vi "BCU诊断标定.vi"(8 "CAN端口":u16(ring), 9 "设备索引号":u16(ring), 10 "CAN卡类型":u32(ring)=21, 11 "Myindex":dbl=1.0) -> (3 "成功":bool)   [LabVIEW 2013] (continued)
                tunnel: w6103 -> [w6106 w6114]
                frame #0 {
                  n4263 = dll-call lib="PTH1abs FBluewave New EnergySVN_WorkAutoTest_TestStandtrunkAutoTest_TestStandDriverZlgCanBHN01è¯»ååæ°data\nkerneldlls\nusbcan.dll" fn="VCI_ClearBuffer"("DeviceType"=w6108, "DeviceInd"=w6107, "CANInd"=w6106) -> (error out=w6109:errorcluster)  [unwired: 4 in, 4 out]
                  n4264 = call <vilib>:"Clear Errors.vi"("error in (no error)"=w6109) -> ()  [unwired: 6 in, 1 out]
                }
                frame #1 {
                  w6113 = u8 137 ("命令")
                  w6112 = u32 1 ("命令序号")
                  n4265 = local read "从板板号"() -> (w6110:u8)
                  n4266 = local write "命令"(w6113) -> ()
                  n4267 = call "多帧发送机制(EV05).vi"("can卡类型"=w6116, "设备索引号"=w6115, "CAN端口"=w6114, "命令"=w6113, "板号"=w6110, "命令序号"=w6112, "输入数据"=dbl[] [0.0]) -> ()  [unwired: 2 in, 11 out]
                  n4268 = local write "命令序号"(w6112) -> ()
                }
              }
            }
            frame #1 {
              n4269 = while {
                tunnel: [w6118] -> w6117
                i -> [w6123]
                stop <- w6120 stop-if-true
                n4270 = global read "EV05全局变量1.vi" "写入超时"() -> (w6118:bool)
                n4271 = Greater Or Equal?(x=w6123, y=25) -> (x >= y?=w6121:bool)
                n4272 = Or(x=w6118, y=w6121) -> (x .or. y?=w6120:bool)
                n4273 = Wait Until Next ms Multiple(millisecond multiple=u32 100 ("毫秒倍数")) -> ()  [unwired: 1 out]
              }
            }
            frame #2 {
              n4274 = case shown="假" w6124 {
                frame False {
                  n4275 = control-ref of="结果"() -> (w6126:refnum<vi>)
                  n4276 = Concatenate Strings("项目软件版本" ("字符串"), "     读取失败" ("字符串")) -> (w6129:string)
                  n4277 = Build Array(w6129) -> (w6128:string[])
                  n4278 = call "表格编辑(版本读取).vi"("新元素/子数组"=w6128, "活动单元格:单元格背景色"=u32 16740749, "MCListbox引用句柄"=w6126) -> ()  [unwired: 9 out]
                }
                frame True {
                }
              }
              n4279 = call <vilib>:"Unset Busy.vi"() -> ()  [unwired: 2 in, 10 out]
            }
          }
        }
        frame "读取故障状态" {
          n4280 = stacked-sequence {
            seq-local: [_ w6155 _] -> [_ _ w6162]
            frame #0 {
              n4281 = local read "设备索引号"() -> (w6132:u16)
              n4282 = local read "CAN卡类型"() -> (w6133:u32)
              n4283 = local read "CAN端口"() -> (w6131:u16)
              n4284 = stacked-sequence {
                tunnel: w6133 -> [w6136 w6145]
                tunnel: w6132 -> [w6135 w6144]
                tunnel: w6131 -> [w6134 w6143]
                frame #0 {
                  n4285 = dll-call lib="PTH1abs FBluewave New EnergySVN_WorkAutoTest_TestStandtrunkAutoTest_TestStandDriverZlgCanBHN01è¯»ååæ°data\nkerneldlls\nusbcan.dll" fn="VCI_ClearBuffer"("DeviceType"=w6136, "DeviceInd"=w6135, "CANInd"=w6134) -> (error out=w6137:errorcluster)  [unwired: 4 in, 4 out]
                  n4286 = call <vilib>:"Clear Errors.vi"("error in (no error)"=w6137) -> ()  [unwired: 6 in, 1 out]
                }
                frame #1 {
                  n4287 = local read "从板板号 2"() -> (w6138:u8)
                  n4288 = case shown="1..30" w6138 {
                    tunnel: [u8 133 ("命令") u8 4 ("命令")] -> w6142
                    frame 0, Default {
                    }
                    frame 1..30 {
                    }
                  }
                  n4289 = local read "状态选择"() -> (w6140:T18)
                  n4290 = local write "命令"(w6142) -> ()
                  n4291 = case shown="\"预充电故障,继电器驱动故障\"" w6140 {
                    tunnel: [1 2 3 4 5 6 7] -> w6139
                    frame "电压,内总电压,外总电压,温度,电流,绝缘,系统时钟,充电均衡,放电均衡", Default {
                    }
                    frame "CPU,CPU内部EE存储器,CPU内部FLASH,内部EE存储器,45db存储器" {
                    }
                    frame "CAN检测故障" {
                    }
                    frame "软件故障" {
                    }
                    frame "RS485,RS232检测故障" {
                    }
                    frame "DI,DO,AI,AO检测故障" {
                    }
                    frame "预充电故障,继电器驱动故障" {
                    }
                  }
                  n4292 = call "多帧发送机制(EV05).vi"("can卡类型"=w6145, "设备索引号"=w6144, "CAN端口"=w6143, "命令"=w6142, "板号"=w6138, "命令序号"=w6139, "输入数据"=dbl[] [0.0]) -> ()  [unwired: 2 in, 11 out]
                  n4293 = local write "命令序号"(w6139) -> ()
                }
              }
            }
            frame #1 {
              n4294 = while {
                tunnel: [w6156] -> w6155
                i -> [w6161]
                stop <- w6158 stop-if-true
                n4295 = global read "EV05全局变量1.vi" "写入超时"() -> (w6156:bool)
                n4296 = Greater Or Equal?(x=w6161, y=25) -> (x >= y?=w6159:bool)
                n4297 = Or(x=w6156, y=w6159) -> (x .or. y?=w6158:bool)
                n4298 = Wait Until Next ms Multiple(millisecond multiple=u32 100 ("毫秒倍数")) -> ()  [unwired: 1 out]
              }
            }
            frame #2 {
              n4299 = case shown="真" w6162 {
                frame False {
                  n4300 = Concatenate Strings("故障信息" ("字符串"), "     读取失败" ("字符串")) -> (w6164:string)
                  n4301 = One Button Dialog(message=w6164, button name ("OK")="确定" ("按钮名称（“确定”）")) -> ()  [unwired: 1 out]
                }
                frame True {
                  n4302 = One Button Dialog(message="故障信息读取完成" ("字符串"), button name ("OK")="确定" ("按钮名称（“确定”）")) -> ()  [unwired: 1 out]
                }
              }
              n4303 = call <vilib>:"Unset Busy.vi"() -> ()  [unwired: 2 in, 10 out]
            }
          }
        }
        frame "平台软件版本读取" {
          n4304 = stacked-sequence {
            seq-local: [_ w6184 _] -> [_ _ w6191]
            frame #0 {
              n4305 = local read "设备索引号"() -> (w6171:u16)
              n4306 = local read "CAN卡类型"() -> (w6172:u32)
              n4307 = local read "CAN端口"() -> (w6170:u16)
              n4308 = stacked-sequence {
                tunnel: w6172 -> [w6175 w6183]
                tunnel: w6171 -> [w6174 w6182]
                tunnel: w6170 -> [w6173 w6181]
                tunnel: u8 137 ("命令") -> [_ w6180]
                frame #0 {
                  n4309 = dll-call lib="PTH1abs FBluewave New EnergySVN_WorkAutoTest_TestStandtrunkAutoTest_TestStandDriverZlgCanBHN01è¯»ååæ°data\nkerneldlls\nusbcan.dll" fn="VCI_ClearBuffer"("DeviceType"=w6175, "DeviceInd"=w6174, "CANInd"=w6173) -> (error out=w6176:errorcluster)  [unwired: 4 in, 4 out]
                  n4310 = call <vilib>:"Clear Errors.vi"("error in (no error)"=w6176) -> ()  [unwired: 6 in, 1 out]
                }
                frame #1 {
                  w6179 = u32 2 ("命令序号")
                  n4311 = local read "从板板号"() -> (w6177:u8)
                  n4312 = local write "命令"(w6180) -> ()
                  n4313 = call "多帧发送机制(EV05).vi"("can卡类型"=w6183, "设备索引号"=w6182, "CAN端口"=w6181, "命令"=w6180, "板号"=w6177, "命令序号"=w6179, "输入数据"=dbl[] [0.0]) -> ()  [unwired: 2 in, 11 out]
                  n4314 = local write "命令序号"(w6179) -> ()
                }
              }
            }
            frame #1 {
              n4315 = while {
                tunnel: [w6185] -> w6184
                i -> [w6190]
                stop <- w6187 stop-if-true
                n4316 = global read "EV05全局变量1.vi" "写入超时"() -> (w6185:bool)
                n4317 = Greater Or Equal?(x=w6190, y=25) -> (x >= y?=w6188:bool)
                n4318 = Or(x=w6185, y=w6188) -> (x .or. y?=w6187:bool)
                n4319 = Wait Until Next ms Multiple(millisecond multiple=u32 100 ("毫秒倍数")) -> ()  [unwired: 1 out]
              }
            }
            frame #2 {
              n4320 = case shown="假" w6191 {
                frame False {
                  n4321 = control-ref of="结果"() -> (w6194:refnum<vi>)
                  n4322 = Concatenate Strings("平台软件版本" ("字符串"), "     读取失败" ("字符串")) -> (w6196:string)
                  n4323 = Build Array(w6196) -> (w6193:string[])
                  n4324 = call "表格编辑(版本读取).vi"("新元素/子数组"=w6193, "活动单元格:单元格背景色"=u32 16740749, "MCListbox引用句柄"=w6194) -> ()  [unwired: 9 out]
                }
                frame True {
                }
              }
              n4325 = call <vilib>:"Unset Busy.vi"() -> ()  [unwired: 2 in, 10 out]
            }
          }
        }
        frame "模块软件版本读取" {
          n4326 = local read "从板板号"() -> (w6198:u8)
          n4327 = local read "模块软件版本"() -> (w6199:T1)
          n4328 = case shown="\"全部读取\"" w6199 {
            selector: w6199 -> [w6200 w6244]
            tunnel: w6198 -> [_ w6243]
            frame "BCUMCAL", Default {
              n4329 = stacked-sequence {
                seq-local: [_ _ w6226 _] -> [_ _ _ w6233]
                tunnel: w6200 -> [_ w6206 _ w6234]
                frame #0 {
                  w6205 = FALSE ("写?")
                  n4330 = call <vilib>:"Set Busy.vi"("disable click? (T)"=FALSE) -> ()  [unwired: 3 in, 8 out]
                  n4331 = local write "写?"(w6205) -> ()
                  n4332 = global write "EV05全局变量1.vi" "流控帧 2"(TRUE ("流控帧 2")) -> ()
                  n4333 = global write "EV05全局变量1.vi" "写入超时"(w6205) -> ()
                  n4334 = local write "控制1"(TRUE ("控制1")) -> ()
                  n4335 = local write "消除"(TRUE ("消除")) -> ()
                }
                frame #1 {
                  n4336 = Quotient & Remainder(x=w6206, y=256) -> (x-y*floor(x/y)=w6207:i32, floor(x/y)=w6208:i32)
                  n4337 = Build Array(w6208, w6207, u8 0 ("板号")) -> (w6211:i32[])
                  n4338 = local read "设备索引号"() -> (w6213:u16)
                  n4339 = local read "CAN卡类型"() -> (w6214:u32)
                  n4340 = local read "CAN端口"() -> (w6212:u16)
                  n4341 = stacked-sequence {
                    tunnel: w6214 -> [w6217 w6225]
                    tunnel: w6213 -> [w6216 w6224]
                    tunnel: w6212 -> [w6215 w6223]
                    tunnel: w6211 -> [_ w6222]
                    frame #0 {
                      n4342 = dll-call lib="PTH1abs FBluewave New EnergySVN_WorkAutoTest_TestStandtrunkAutoTest_TestStandDriverZlgCanBHN01è¯»ååæ°data\nkerneldlls\nusbcan.dll" fn="VCI_ClearBuffer"("DeviceType"=w6217, "DeviceInd"=w6216, "CANInd"=w6215) -> (error out=w6218:errorcluster)  [unwired: 4 in, 4 out]
                      n4343 = call <vilib>:"Clear Errors.vi"("error in (no error)"=w6218) -> ()  [unwired: 6 in, 1 out]
                    }
                    frame #1 {
                      w6221 = u8 137 ("命令")
                      w6219 = u32 3 ("命令序号")
                      n4344 = local read "从板板号"() -> (w6220:u8)
                      n4345 = local write "命令"(w6221) -> ()
                      n4346 = call "多帧发送机制(EV05).vi"("can卡类型"=w6225, "设备索引号"=w6224, "CAN端口"=w6223, "命令"=w6221, "板号"=w6220, "命令序号"=w6219, "输入数据"=w6222) -> ()  [unwired: 2 in, 11 out]
                      n4347 = local write "命令序号"(w6219) -> ()
                    }
                  }
                }
                frame #2 {
                  n4348 = while {
                    tunnel: [w6227] -> w6226
                    i -> [w6232]
                    stop <- w6228 stop-if-true
                    n4349 = global read "EV05全局变量1.vi" "写入超时"() -> (w6227:bool)
                    n4350 = Greater Or Equal?(x=w6232, y=25) -> (x >= y?=w6229:bool)
                    n4351 = Or(x=w6227, y=w6229) -> (x .or. y?=w6228:bool)
                    n4352 = Wait Until Next ms Multiple(millisecond multiple=u32 100 ("毫秒倍数")) -> ()  [unwired: 1 out]
                  }
                }
                frame #3 {
                  n4353 = call <vilib>:"Unset Busy.vi"() -> ()  [unwired: 2 in, 10 out]
                  n4354 = case shown="假" w6233 {
                    tunnel: w6234 -> [w6236 _]
                    frame False {
                      n4355 = Number To Decimal String(number=w6236) -> (decimal integer string=w6237:string)  [unwired: 1 out]
                      n4356 = control-ref of="结果"() -> (w6238:refnum<vi>)
                      n4357 = Concatenate Strings("模块" ("字符串"), w6237, "     读取失败" ("字符串")) -> (w6241:string)
                      n4358 = Build Array(w6241) -> (w6240:string[])
                      n4359 = call "表格编辑(版本读取).vi"("新元素/子数组"=w6240, "活动单元格:单元格背景色"=u32 16740749, "MCListbox引用句柄"=w6238) -> ()  [unwired: 9 out]
                    }
                    frame True {
                    }
                  }
                }
              }
            }
            frame "全部读取" {
              n4360 = stacked-sequence {
                seq-local: [w6245 _] -> [_ w6283]
                tunnel: w6244 -> [_ w6285]
                tunnel: w6243 -> [w6246 w6284]
                frame #0 {
                  n4361 = stacked-sequence {
                    tunnel: w6246 -> [_ w6255 _]
                    tunnel: [_ _ w6275] -> w6245
                    frame #0 {
                      w6251 = FALSE ("写?")
                      n4362 = control-ref of="模块软件版本 2"() -> (w6249:refnum<vi>)
                      n4363 = call <vilib>:"Set Busy.vi"("disable click? (T)"=FALSE) -> ()  [unwired: 3 in, 8 out]
                      n4364 = local write "写?"(w6251) -> ()
                      n4365 = property class="MCListbox (严格)"(reference=w6249, "ItemNames"=string[][] []) -> ()  [unwired: 1 in, 2 out]
                      n4366 = global write "EV05全局变量1.vi" "写入超时"(w6251) -> ()
                      n4367 = local write "消除"(TRUE ("消除")) -> ()
                      n4368 = local write "控制1"(TRUE ("控制1")) -> ()
                      n4369 = global write "EV05全局变量1.vi" "流控帧 2"(TRUE ("流控帧 2")) -> ()
                      n4370 = local write "MODEL号"(u8[] [] ("MODEL号")) -> ()
                    }
                    frame #1 {
                      n4371 = local read "设备索引号"() -> (w6257:u16)
                      n4372 = local read "CAN卡类型"() -> (w6258:u32)
                      n4373 = local read "CAN端口"() -> (w6256:u16)
                      n4374 = stacked-sequence {
                        tunnel: w6258 -> [w6261 w6274]
                        tunnel: w6257 -> [w6260 w6273]
                        tunnel: w6256 -> [w6259 w6272]
                        tunnel: w6255 -> [_ w6264]
                        frame #0 {
                          n4375 = dll-call lib="PTH1abs FBluewave New EnergySVN_WorkAutoTest_TestStandtrunkAutoTest_TestStandDriverZlgCanBHN01è¯»ååæ°data\nkerneldlls\nusbcan.dll" fn="VCI_ClearBuffer"("DeviceType"=w6261, "DeviceInd"=w6260, "CANInd"=w6259) -> (error out=w6262:errorcluster)  [unwired: 4 in, 4 out]
                          n4376 = call <vilib>:"Clear Errors.vi"("error in (no error)"=w6262) -> ()  [unwired: 6 in, 1 out]
                        }
                        frame #1 {
                          w6270 = u8 137 ("命令")
                          w6268 = u32 3 ("命令序号")
                          n4377 = Quotient & Remainder(x=u8 0 ("板号"), y=256) -> (x-y*floor(x/y)=w6265:i32, floor(x/y)=w6266:i32)
                          n4378 = local write "命令"(w6270) -> ()
                          n4379 = Build Array(w6266, w6265, u8 0 ("板号")) -> (w6271:i32[])
                          n4380 = call "多帧发送机制(EV05).vi"("can卡类型"=w6274, "设备索引号"=w6273, "CAN端口"=w6272, "命令"=w6270, "板号"=w6264, "命令序号"=w6268, "输入数据"=w6271) -> ()  [unwired: 2 in, 11 out]
                          n4381 = local write "命令序号"(w6268) -> ()
                        }
                      }
                    }
                    frame #2 {
                      n4382 = while {
                        tunnel: [w6277] -> w6275
                        i -> [w6281]
                        stop <- w6278 stop-if-true
                        n4383 = local read "强制停止版本读取"() -> (w6276:bool)
                        n4384 = global read "EV05全局变量1.vi" "写入超时"() -> (w6277:bool)
                        n4385 = Greater Or Equal?(x=w6281, y=35) -> (x >= y?=w6279:bool)
                        n4386 = Compound Arithmetic op=OR(w6276, w6277, w6279) -> (w6278:bool)
                        n4387 = Wait Until Next ms Multiple(millisecond multiple=u32 100 ("毫秒倍数")) -> ()  [unwired: 1 out]
                      }
                    }
                  }
                }
                frame #1 {
                  n4388 = case shown="真" w6283 {
                    tunnel: w6285 -> [_ w6295]
                    tunnel: w6284 -> [_ w6294]
                    frame False {
                      n4389 = control-ref of="结果"() -> (w6287:refnum<vi>)
                      n4390 = Concatenate Strings("模块编号" ("字符串"), "读取失败" ("字符串")) -> (w6290:string)
                      n4391 = Build Array(w6290) -> (w6289:string[])
                      n4392 = call "表格编辑(版本读取).vi"("新元素/子数组"=w6289, "活动单元格:单元格背景色"=u32 16740749, "MCListbox引用句柄"=w6287) -> ()  [unwired: 9 out]
                      n4393 = call <vilib>:"Unset Busy.vi"() -> ()  [unwired: 11 in, 1 out]
                    }
                    frame True {
                      n4394 = local read "MODEL号"() -> (w6293:u8[])
                      n4395 = Array Size(array=w6293) -> (size(s)=w6292:i32)
                      n4396 = for {
                        tunnel: w6295 -> [_]
                        tunnel: w6294 -> [w6298]
                        tunnel: w6293 -> [w6297] mode=indexing
                        tunnel: w6292 -> [w6296]
                        i -> [w6300]
                        n4397 = Increment(x=w6300) -> (x+1=w6299:i32)
                        n4398 = stacked-sequence {
                          seq-local: [_ _ _ w6327 _ _] -> [_ _ _ _ w6336 _]
                          seq-local: [_ w6306 _ _ _ _] -> [_ _ _ _ w6335 _]
                          tunnel: w6299 -> [_ _ _ _ _ w6347]
                          tunnel: w6297 -> [_ w6306 _ _ _ _]
                          tunnel: w6298 -> [_ w6307 _ _ _ _]
                          tunnel: w6296 -> [_ _ _ _ _ w6345]
                          frame #0 {
                            w6302 = FALSE ("写?")
                            n4399 = call <vilib>:"Set Busy.vi"("disable click? (T)"=FALSE) -> ()  [unwired: 3 in, 8 out]
                            n4400 = local write "写?"(w6302) -> ()
                            n4401 = global write "EV05全局变量1.vi" "写入超时"(w6302) -> ()
                            n4402 = global write "EV05全局变量1.vi" "流控帧 2"(TRUE ("流控帧 2")) -> ()
                            n4403 = local write "控制1"(TRUE ("控制1")) -> ()
                            n4404 = local write "消除"(TRUE ("消除")) -> ()
                          }
                          frame #1 {
                            n4405 = local read "设备索引号"() -> (w6309:u16)
                            n4406 = local read "CAN卡类型"() -> (w6310:u32)
                            n4407 = local read "CAN端口"() -> (w6308:u16)
                            n4408 = stacked-sequence {
                              tunnel: w6310 -> [w6313 w6326]
                              tunnel: w6309 -> [w6312 w6325]
                              tunnel: w6308 -> [w6311 w6324]
                              tunnel: w6307 -> [_ w6316]
                              tunnel: w6306 -> [_ w6315]
                              frame #0 {
                                n4409 = dll-call lib="PTH1abs FBluewave New EnergySVN_WorkAutoTest_TestStandtrunkAutoTest_TestStandDriverZlgCanBHN01è¯»ååæ°data\nkerneldlls\nusbcan.dll" fn="VCI_ClearBuffer"("DeviceType"=w6313, "DeviceInd"=w6312, "CANInd"=w6311) -> (error out=w6314:errorcluster)  [unwired: 4 in, 4 out]
                                n4410 = call <vilib>:"Clear Errors.vi"("error in (no error)"=w6314) -> ()  [unwired: 6 in, 1 out]
                              }
                              frame #1 {
                                w6322 = u8 137 ("命令")
                                w6320 = u32 3 ("命令序号")
                                n4411 = Quotient & Remainder(x=w6315, y=256) -> (x-y*floor(x/y)=w6317:i32, floor(x/y)=w6318:i32)
                                n4412 = local write "命令"(w6322) -> ()
                                n4413 = Build Array(w6318, w6317, u8 0 ("板号")) -> (w6323:i32[])
                                n4414 = call "多帧发送机制(EV05).vi"("can卡类型"=w6326, "设备索引号"=w6325, "CAN端口"=w6324, "命令"=w6322, "板号"=w6316, "命令序号"=w6320, "输入数据"=w6323) -> ()  [unwired: 2 in, 11 out]
                                n4415 = local write "命令序号"(w6320) -> ()
                              }
                            }
                          }
                          frame #2 {
                          }
                          frame #3 {
                            n4416 = while {
                              tunnel: [w6329] -> w6327
                              i -> [w6333]
                              stop <- w6330 stop-if-true
                              n4417 = local read "强制停止版本读取"() -> (w6328:bool)
                              n4418 = global read "EV05全局变量1.vi" "写入超时"() -> (w6329:bool)
                              n4419 = Greater Or Equal?(x=w6333, y=25) -> (x >= y?=w6331:bool)
                              n4420 = Compound Arithmetic op=OR(w6328, w6329, w6331) -> (w6330:bool)
                              n4421 = Wait Until Next ms Multiple(millisecond multiple=u32 100 ("毫秒倍数")) -> ()  [unwired: 1 out]
                            }
                          }
                          frame #4 {
                            n4422 = call <vilib>:"Unset Busy.vi"() -> ()  [unwired: 11 in, 1 out]
                            n4423 = case shown="假" w6336 {
                              tunnel: w6335 -> [w6338 _]
                              frame False {
                                n4424 = control-ref of="结果"() -> (w6340:refnum<vi>)
                                n4425 = Number To Decimal String(number=w6338) -> (decimal integer string=w6339:string)  [unwired: 1 out]
                                n4426 = Concatenate Strings("模块" ("字符串"), w6339, "     读取失败" ("字符串")) -> (w6343:string)
                                n4427 = Build Array(w6343) -> (w6342:string[])
                                n4428 = call "表格编辑(版本读取).vi"("新元素/子数组"=w6342, "活动单元格:单元格背景色"=u32 16740749, "MCListbox引用句柄"=w6340) -> ()  [unwired: 9 out]
                              }
                              frame True {
                              }
                            }
                          }
                          frame #5 {
                            n4429 = Equal?(x=w6345, y=w6347) -> (x = y?=w6346:bool)
                            n4430 = case shown="真" w6346 {
                              frame False {
                              }
                              frame True {
                                n4431 = control-ref of="模块软件版本 2"() -> (w6358:refnum<vi>)
                                n4432 = local read "模块版本名称"() -> (w6357:string[][])
                                n4433 = local read "模块版本值"() -> (w6353:string[][])
                                n4434 = control-ref of="结果"() -> (w6365:refnum<vi>)
                                n4435 = property class="MCListbox (严格)"(reference=w6358) -> ("ItemNames"=w6361:string[][])  [unwired: 1 in, 2 out]
                                n4436 = local read "从板板号"() -> (w6348:u8)
                                n4437 = Concatenate Strings("模块版本读取完成" ("字符串")) -> (w6368:string)
                                n4438 = Build Array(w6368) -> (w6367:string[])
                                n4439 = call "表格编辑(版本读取).vi"("新元素/子数组"=w6367, "活动单元格:单元格背景色"=u32 21937, "MCListbox引用句柄"=w6365) -> ()  [unwired: 9 out]
                                n4440 = Transpose 2D Array(2D array=w6361) -> (transposed array=w6362:string[][])
                                n4441 = local write "强制停止版本读取"(FALSE ("强制停止 2")) -> ()
                                n4442 = local read "模块个数"() -> (w6351:u8[])
                                n4443 = Index Array(array=w6362, index (row) #1=0 ("索引 (行)"), index (row) #2=1 ("索引 (行)")) -> (element #1=w6352:string[], element #2=w6354:string[])  [unwired: 2 in]
                                n4444 = Replace Array Subset(array=w6357, new element=w6352, index (row)=w6348) -> (w6356:string[][])  [unwired: 1 in]
                                n4445 = Replace Array Subset(array=w6353, new element=w6354, index (row)=w6348) -> (w6355:string[][])  [unwired: 1 in]
                                n4446 = local write "模块版本名称"(w6356) -> ()
                                n4447 = local write "模块版本值"(w6355) -> ()
                                n4448 = Array Size(array=w6352) -> (size(s)=w6349:i32)
                                n4449 = Replace Array Subset(array=w6351, new element=w6349, index=w6348) -> (w6350:u8[])
                                n4450 = local write "模块个数"(w6350) -> ()
                              }
                            }
                          }
                        }
                      }
                    }
                  }
                }
              }
            }
          }
        }
        frame "硬件版本读取" {
          n4451 = stacked-sequence {
            seq-local: [_ _ w6376 _] -> [_ _ _ w6383]
            frame #0 {
              w6372 = u8 137 ("命令")
              w6371 = u32 4 ("命令序号")
              n4452 = local read "设备索引号"() -> (w6374:u16)
              n4453 = local read "CAN卡类型"() -> (w6375:u32)
              n4454 = local read "CAN端口"() -> (w6373:u16)
              n4455 = local read "从板板号"() -> (w6369:u8)
              n4456 = local write "命令"(w6372) -> ()
              n4457 = call "多帧发送机制(EV05).vi"("can卡类型"=w6375, "设备索引号"=w6374, "CAN端口"=w6373, "命令"=w6372, "板号"=w6369, "命令序号"=w6371, "输入数据"=dbl[] [0.0]) -> ()  [unwired: 2 in, 11 out]
              n4458 = local write "命令序号"(w6371) -> ()
            }
            frame #1 {
            }
            frame #2 {
              n4459 = while {
                tunnel: [w6377] -> w6376
                i -> [w6382]
                stop <- w6378 stop-if-true
                n4460 = global read "EV05全局变量1.vi" "写入超时"() -> (w6377:bool)
                n4461 = Greater Or Equal?(x=w6382, y=25) -> (x >= y?=w6379:bool)
                n4462 = Or(x=w6377, y=w6379) -> (x .or. y?=w6378:bool)
                n4463 = Wait Until Next ms Multiple(millisecond multiple=u32 100 ("毫秒倍数")) -> ()  [unwired: 1 out]
              }
            }
            frame #3 {
              n4464 = case shown="假" w6383 {
                frame False {
                  n4465 = control-ref of="结果"() -> (w6385:refnum<vi>)
                  n4466 = Concatenate Strings("硬件版本" ("字符串"), "     读取失败" ("字符串")) -> (w6388:string)
                  n4467 = Build Array(w6388) -> (w6387:string[])
                  n4468 = call "表格编辑(版本读取).vi"("新元素/子数组"=w6387, "活动单元格:单元格背景色"=u32 16740749, "MCListbox引用句柄"=w6385) -> ()  [unwired: 9 out]
                }
                frame True {
                }
              }
              n4469 = call <vilib>:"Unset Busy.vi"() -> ()  [unwired: 2 in, 10 out]
            }
          }
        }
        frame "写配置文件" {
          n4470 = disable-structure shown="启用" {
            frame Enabled {
              n4471 = local read "主从选择"() -> (w6396:enum32{"主板", "从板"})
              n4472 = case shown="\"从板\"" w6396 {
                tunnel: [w6415 w6606] -> w6399
                tunnel: ["M0" w6612] -> w6397
                frame "主板", Default {
                  n4473 = stacked-sequence {
                    seq-local: [w6429 _ _ _ _ _ _] -> [_ w6458 _ _ _ _ _]
                    seq-local: [string[] ["电池额定容量", "电池实际容量", "SOC", "SOH", "车牌号", "配置文件版本", "产品编号", "系统时钟"] _ _ _ _ _ _] -> [_ w6453 _ _ _ _ _]
                    seq-local: [_ _ _ _ string[] ["风机开启温度", "风机关闭温度", "加热开启温度", "加热关闭温度", "风机开启温差", "风机关闭温差", "加热关闭温差"] _ _] -> [_ _ _ _ _ w6558 _]
                    seq-local: [_ _ _ _ w6539 _ _] -> [_ _ _ _ _ w6556 _]
                    tunnel: [w6430 _ _ _ _ _ _] -> w6417
                    tunnel: [_ w6460 _ _ _ _ _] -> w6414
                    tunnel: [_ _ w6484 _ _ _ _] -> w6413
                    tunnel: [_ _ _ w6511 _ _ _] -> w6412
                    tunnel: [_ _ _ _ _ w6559 _] -> w6411
                    tunnel: [_ _ _ _ _ _ w6576] -> w6410
                    frame #0 {
                      w6421 = string[] ["", "", "", "", "", "", "", "", "", "", "  "]
                      n4474 = control-ref of="项目信息"() -> (w6449:refnum<vi>)
                      n4475 = property class="Tbl (严格)"(reference=w6449) -> ("Value"=w6425:string[][])  [unwired: 1 in, 2 out]
                      n4476 = control-ref of="项目信息2"() -> (w6443:refnum<vi>)
                      n4477 = Index Array(array=w6425, index (col)=0 ("禁用的索引 (列)")) -> (element=w6426:string[])  [unwired: 1 in]
                      n4478 = property class="Clust (严格)"(reference=w6443) -> ("Value"=w6442:T9)  [unwired: 1 in, 2 out]
                      n4479 = Index Array(array=w6425, index (col)=1 ("禁用的索引 (列)")) -> (element=w6424:string[])  [unwired: 1 in]
                      n4480 = local read "从板个数"() -> (w6448:dbl)
                      n4481 = Number To Decimal String(number=w6448) -> (decimal integer string=w6447:string)  [unwired: 1 out]
                      n4482 = Insert Into Array(array=w6426, new element=w6421) -> (w6423:string[])  [unwired: 1 in]
                      n4483 = Insert Into Array(array=w6424, new element=w6421) -> (w6422:string[])  [unwired: 1 in]
                      n4484 = Unbundle(w6442) -> ("电池额定容量(A)"=w6441:dbl, "电池实际容量(A)"=w6440:dbl, "车架(牌)号"=w6438:string, "配置文件版本"=w6437:string, "SOH(%)"=w6432:dbl, "SOC(%)"=w6431:dbl, "产品编号"=w6436:string, "系统时钟"=w6435:string)  [unwired: 1 out]
                      n4485 = Build Array("从板个数" ("元素"), w6447) -> (w6444:string[])
                      n4486 = Build Array(w6423, w6422) -> (w6419:string[][])
                      n4487 = Transpose 2D Array(2D array=w6419) -> (transposed array=w6418:string[][])
                      n4488 = Build Array(w6441, w6440, w6431, w6432) -> (w6439:dbl[])
                      n4489 = Build Array(w6438, w6437, w6436, w6435) -> (w6433:string[])
                      n4490 = for {
                        tunnel: w6439 -> [w6451] mode=indexing
                        tunnel: [w6450] -> w6434 mode=indexing
                        n4491 = Format Into String(format string="%#f" ("格式字符串"), w6451) -> (resulting string=w6450:string)  [unwired: 2 in, 1 out]
                      }
                      n4492 = Insert Into Array(array=w6418, index (row)=0 ("索引 (行)"), new element=w6444) -> (w6430:string[][])  [unwired: 1 in]
                      n4493 = Insert Into Array(array=w6434, new element=w6433) -> (w6429:string[])  [unwired: 1 in]
                    }
                    frame #1 {
                      n4494 = control-ref of="一级故障"() -> (w6480:refnum<vi>)
                      n4495 = property class="Clust (严格)"(reference=w6480) -> ("Value"=w6479:T10)  [unwired: 1 in, 2 out]
                      n4496 = Unbundle(w6479) -> ("总电压过高"=w6478:dbl, "整组电压不均衡"=w6473:dbl, "SOC过高"=w6466:dbl, "单体电压过高"=w6469:dbl, "总电压过低"=w6477:dbl, "温度过高"=w6476:dbl, "温度过低"=w6475:dbl, "单组电压不均衡"=w6474:dbl, "整组温度不均衡"=w6471:dbl, "单组温度不均衡"=w6472:dbl, "单体电压过低"=w6470:dbl, "充电电流过高"=w6468:dbl, "放电电流过高"=w6467:dbl, "SOC过低"=w6465:dbl, "内阻过大"=w6464:dbl, "极柱温度过高"=w6463:dbl, "SOH过低"=w6462:dbl)
                      n4497 = Build Array(w6478, w6477, w6476, w6475, w6474, w6473, w6472, w6471, w6469, w6470, w6468, w6467, w6466, w6465, w6464, w6463, w6462) -> (w6461:dbl[])
                      n4498 = for {
                        tunnel: w6461 -> [w6482] mode=indexing
                        tunnel: [w6481] -> w6457 mode=indexing
                        n4499 = Format Into String(format string="%#f" ("格式字符串"), w6482) -> (resulting string=w6481:string)  [unwired: 2 in, 1 out]
                      }
                      n4500 = Insert Into Array(array=w6458, new element=w6457) -> (w6456:string[])  [unwired: 1 in]
                      n4501 = Insert Into Array(array=w6453, new element=string[] ["总电压过高一级", "总电压过低一级", "温度过高一级", "温度过低一级", "单组电压不均衡一级", "整组电压不均衡一级", "单组温度不均衡一级", "整组温度不均衡一级", "单体电压过高一级", "单体电压过低一级", "充电电流过高一级", "放电电流过高一级", "SOC过高一级", "SOC过低一级", "内阻过大一级", "极柱温度过高一级", "SOH过低一级"]) -> (w6455:string[])  [unwired: 1 in]
                      n4502 = Build Array(w6455, w6456) -> (w6454:string[][])
                      n4503 = Transpose 2D Array(2D array=w6454) -> (transposed array=w6460:string[][])
                    }
                    frame #2 {
                      n4504 = control-ref of="一级故障 2"() -> (w6485:refnum<vi>)
                      n4505 = property class="Clust (严格)"(reference=w6485) -> ("Value"=w6507:T10)  [unwired: 1 in, 2 out]
                      n4506 = Unbundle(w6507) -> ("总电压过高"=w6506:dbl, "整组电压不均衡"=w6501:dbl, "SOC过高"=w6494:dbl, "单体电压过高"=w6497:dbl, "总电压过低"=w6505:dbl, "温度过高"=w6504:dbl, "温度过低"=w6503:dbl, "单组电压不均衡"=w6502:dbl, "整组温度不均衡"=w6499:dbl, "单组温度不均衡"=w6500:dbl, "单体电压过低"=w6498:dbl, "充电电流过高"=w6496:dbl, "放电电流过高"=w6495:dbl, "SOC过低"=w6493:dbl, "内阻过大"=w6492:dbl, "极柱温度过高"=w6491:dbl, "SOH过低"=w6490:dbl)
                      n4507 = Build Array(w6506, w6505, w6504, w6503, w6502, w6501, w6500, w6499, w6497, w6498, w6496, w6495, w6494, w6493, w6492, w6491, w6490) -> (w6489:dbl[])
                      n4508 = for {
                        tunnel: w6489 -> [w6509] mode=indexing
                        tunnel: [w6508] -> w6488 mode=indexing
                        n4509 = Format Into String(format string="%#f" ("格式字符串"), w6509) -> (resulting string=w6508:string)  [unwired: 2 in, 1 out]
                      }
                      n4510 = Build Array(string[] ["总电压过高二级", "总电压过低二级", "温度过高二级", "温度过低二级", "单组电压不均衡二级", "整组电压不均衡二级", "单组温度不均衡二级", "整组温度不均衡二级", "单体电压过高二级", "单体电压过低二级", "充电电流过高二级", "放电电流过高二级", "SOC过高二级", "SOC过低二级", "内阻过大二级", "极柱温度过高二级", "SOH过低二级"], w6488) -> (w6486:string[][])
                      n4511 = Transpose 2D Array(2D array=w6486) -> (transposed array=w6484:string[][])
                    }
                    frame #3 {
                      n4512 = control-ref of="一级故障 3"() -> (w6512:refnum<vi>)
                      n4513 = property class="Clust (严格)"(reference=w6512) -> ("Value"=w6534:T10)  [unwired: 1 in, 2 out]
                      n4514 = Unbundle(w6534) -> ("总电压过高"=w6533:dbl, "整组电压不均衡"=w6528:dbl, "SOC过高"=w6521:dbl, "单体电压过高"=w6524:dbl, "总电压过低"=w6532:dbl, "温度过高"=w6531:dbl, "温度过低"=w6530:dbl, "单组电压不均衡"=w6529:dbl, "整组温度不均衡"=w6526:dbl, "单组温度不均衡"=w6527:dbl, "单体电压过低"=w6525:dbl, "充电电流过高"=w6523:dbl, "放电电流过高"=w6522:dbl, "SOC过低"=w6520:dbl, "内阻过大"=w6519:dbl, "极柱温度过高"=w6518:dbl, "SOH过低"=w6517:dbl)
                      n4515 = Build Array(w6533, w6532, w6531, w6530, w6529, w6528, w6527, w6526, w6524, w6525, w6523, w6522, w6521, w6520, w6519, w6518, w6517) -> (w6516:dbl[])
                      n4516 = for {
                        tunnel: w6516 -> [w6536] mode=indexing
                        tunnel: [w6535] -> w6515 mode=indexing
                        n4517 = Format Into String(format string="%#f" ("格式字符串"), w6536) -> (resulting string=w6535:string)  [unwired: 2 in, 1 out]
                      }
                      n4518 = Build Array(string[] ["总电压过高三级", "总电压过低三级", "温度过高三级", "温度过低三级", "单组电压不均衡三级", "整组电压不均衡三级", "单组温度不均衡三级", "整组温度不均衡三级", "单体电压过高三级", "单体电压过低三级", "充电电流过高三级", "放电电流过高三级", "SOC过高三级", "SOC过低三级", "内阻过大三级", "极柱温度过高三级", "SOH过低三级"], w6515) -> (w6513:string[][])
                      n4519 = Transpose 2D Array(2D array=w6513) -> (transposed array=w6511:string[][])
                    }
                    frame #4 {
                      n4520 = control-ref of="加热控制参数"() -> (w6549:refnum<vi>)
                      n4521 = property class="Clust (严格)"(reference=w6549) -> ("Value"=w6548:T11)  [unwired: 1 in, 2 out]
                      n4522 = Unbundle(w6548) -> ("风机开启温度"=w6547:dbl, "风机关闭温度"=w6546:dbl, "加热开启温度"=w6545:dbl, "加热关闭温度"=w6544:dbl, "风机开启温差"=w6543:dbl, "风机关闭温差"=w6542:dbl, "加热关闭温差"=w6538:dbl)
                      n4523 = Build Array(w6547, w6546, w6545, w6544, w6543, w6542, w6538) -> (w6541:dbl[])
                      n4524 = for {
                        tunnel: w6541 -> [w6551] mode=indexing
                        tunnel: [w6550] -> w6539 mode=indexing
                        n4525 = Format Into String(format string="%#f" ("格式字符串"), w6551) -> (resulting string=w6550:string)  [unwired: 2 in, 1 out]
                      }
                    }
                    frame #5 {
                      n4526 = control-ref of="充电控制参数"() -> (w6569:refnum<vi>)
                      n4527 = property class="Clust (严格)"(reference=w6569) -> ("Value"=w6571:T12)  [unwired: 1 in, 2 out]
                      n4528 = Unbundle(w6571) -> ("最大允许单体电压"=w6568:dbl, "最大允许总电压"=w6567:dbl, "最小允许单体电压"=w6566:dbl, "最大允许充电电流"=w6565:dbl, "最小允许充电电流"=w6564:dbl, "最大允许充电温度"=w6563:dbl, "最小允许充电温度"=w6562:dbl, "电流步长"=w6561:dbl)
                      n4529 = Build Array(w6568, w6567, w6566, w6565, w6564, w6563, w6562, w6561) -> (w6570:dbl[])
                      n4530 = for {
                        tunnel: w6570 -> [w6573] mode=indexing
                        tunnel: [w6572] -> w6555 mode=indexing
                        n4531 = Format Into String(format string="%#f" ("格式字符串"), w6573) -> (resulting string=w6572:string)  [unwired: 2 in, 1 out]
                      }
                      n4532 = Insert Into Array(array=w6556, new element=w6555) -> (w6554:string[])  [unwired: 1 in]
                      n4533 = Insert Into Array(array=w6558, new element=string[] ["最大允许单体电压", "最大允许总电压", "最小允许单体电压", "最大允许充电电流", "最小允许充电电流", "最大允许充电温度", "最小允许充电温度", "电流步长"]) -> (w6553:string[])  [unwired: 1 in]
                      n4534 = Build Array(w6553, w6554) -> (w6560:string[][])
                      n4535 = Transpose 2D Array(2D array=w6560) -> (transposed array=w6559:string[][])
                    }
                    frame #6 {
                      n4536 = control-ref of="电池信息"() -> (w6597:refnum<vi>)
                      n4537 = property class="Clust (严格)"(reference=w6597) -> ("Value"=w6600:T13)  [unwired: 1 in, 2 out]
                      n4538 = Unbundle(w6600) -> ("电池串联"=w6596:dbl, "电池并联"=w6595:dbl, "累计放电总安时"=w6593:dbl, "电池包额定容量"=w6592:dbl, "电池包额定能量(kWh)"=w6591:dbl, "电池包额定总电压"=w6590:dbl, "累计充电总安时"=w6594:dbl, "电池充满次数"=w6589:dbl, "电池放空次数"=w6588:dbl, "电池充电次数"=w6587:dbl, "电池生产日期"=w6585:string, "电池厂家"=w6584:string, "电池类型"=w6583:string, "电池包组号"=w6582:string, "电池包产权标识"=w6581:string, "电池应用车型"=w6580:string, "实际容量"=w6575:dbl)
                      n4539 = Build Array(w6585, w6584, w6583, w6582, w6581, w6580) -> (w6579:string[])
                      n4540 = Build Array(w6596, w6595, w6594, w6593, w6592, w6591, w6590, w6589, w6588, w6587, w6575) -> (w6586:dbl[])
                      n4541 = for {
                        tunnel: w6586 -> [w6602] mode=indexing
                        tunnel: [w6601] -> w6578 mode=indexing
                        n4542 = Format Into String(format string="%#f" ("格式字符串"), w6602) -> (resulting string=w6601:string)  [unwired: 2 in, 1 out]
                      }
                      n4543 = Insert Into Array(array=w6579, new element=w6578) -> (w6577:string[])  [unwired: 1 in]
                      n4544 = call <vilib>:"Unset Busy.vi"() -> ()  [unwired: 2 in, 10 out]
                      n4545 = Build Array(string[] ["电池生产日期", "电池厂商", "电池类型", "电池包组号", "电池包产权标识", "电池包应用车型", "电池串联", "电池并联", "累计充电总安时", "累计放电总安时", "电池包额定容量", "电池包额定能量", "电池包额定总电压", "电池充满次数", "电池放空次数", "电池充电次数", "实际容量"], w6577) -> (w6598:string[][])
                      n4546 = Transpose 2D Array(2D array=w6598) -> (transposed array=w6576:string[][])
                    }
                  }
                  n4547 = Insert Into Array(array=w6417, index (col)=2 ("禁用的索引 (列)"), new element #1=w6414, new element #2=w6413, new element #3=w6412, new element #4=w6411, new element #5=w6410) -> (w6415:string[][])  [unwired: 1 in]
                }
                frame "从板" {
                  n4548 = local read "从板号"() -> (w6614:u8)
                  n4549 = Number To Decimal String(number=w6614) -> (decimal integer string=w6611:string)  [unwired: 1 out]
                  n4550 = Concatenate Strings("S", w6611) -> (w6612:string)
                  n4551 = Build Array("从板号" ("元素"), w6611) -> (w6609:string[])
                  n4552 = stacked-sequence {
                    seq-local: [string[] ["风机开启温度", "风机关闭温度", "加热开启温度", "加热关闭温度", "风机开启温差", "风机关闭温差", "加热关闭温差"] _ _ _ _ _] -> [_ _ _ w6683 _ _]
                    seq-local: [w6626 _ _ _ _ _] -> [_ _ _ w6679 _ _]
                    seq-local: [_ string[] ["电压过高一级", "电压过低一级", "温度过高一级", "温度过低一级", "电压不均衡一级", "温度不均衡一级", "SOC过低一级"] _ _ _ _] -> [_ _ _ w6682 _ _]
                    seq-local: [_ w6644 _ _ _ _] -> [_ _ _ w6678 _ _]
                    seq-local: [_ _ string[] ["电压过高二级", "电压过低二级", "温度过高二级", "温度过低二级", "电压不均衡二级", "温度不均衡二级", "SOC过低二级"] _ _ _] -> [_ _ _ w6681 _ _]
                    seq-local: [_ _ w6659 _ _ _] -> [_ _ _ w6677 _ _]
                    tunnel: w6609 -> [w6639 _ _ _ _ _]
                    tunnel: [w6628 _ _ _ _ _] -> w6607
                    tunnel: [_ _ _ w6684 _ _] -> w6605
                    tunnel: [_ _ _ _ w6722 _] -> w6604
                    tunnel: [_ _ _ _ _ w6758] -> _
                    frame #0 {
                      w6619 = string[] ["", "", "", "", "", "", "", "", "", "", "  "]
                      n4553 = control-ref of="项目信息 2"() -> (w6638:refnum<vi>)
                      n4554 = property class="Tbl (严格)"(reference=w6638) -> ("Value"=w6616:string[][])  [unwired: 1 in, 2 out]
                      n4555 = control-ref of="加热控制参数"() -> (w6630:refnum<vi>)
                      n4556 = property class="Clust (严格)"(reference=w6630) -> ("Value"=w6637:T11)  [unwired: 1 in, 2 out]
                      n4557 = Unbundle(w6637) -> ("风机开启温度"=w6636:dbl, "风机关闭温度"=w6635:dbl, "加热开启温度"=w6634:dbl, "加热关闭温度"=w6633:dbl, "风机开启温差"=w6632:dbl, "风机关闭温差"=w6631:dbl, "加热关闭温差"=w6625:dbl)
                      n4558 = Build Array(w6636, w6635, w6634, w6633, w6632, w6631, w6625) -> (w6629:dbl[])
                      n4559 = for {
                        tunnel: w6629 -> [w6642] mode=indexing
                        tunnel: [w6641] -> w6626 mode=indexing
                        n4560 = Format Into String(format string="%#f" ("格式字符串"), w6642) -> (resulting string=w6641:string)  [unwired: 2 in, 1 out]
                      }
                      n4561 = Index Array(array=w6616, index (col)=0 ("禁用的索引 (列)")) -> (element=w6623:string[])  [unwired: 1 in]
                      n4562 = Index Array(array=w6616, index (col)=1 ("禁用的索引 (列)")) -> (element=w6622:string[])  [unwired: 1 in]
                      n4563 = Insert Into Array(array=w6623, new element=w6619) -> (w6621:string[])  [unwired: 1 in]
                      n4564 = Insert Into Array(array=w6622, new element=w6619) -> (w6620:string[])  [unwired: 1 in]
                      n4565 = Build Array(w6621, w6620) -> (w6617:string[][])
                      n4566 = Transpose 2D Array(2D array=w6617) -> (transposed array=w6615:string[][])
                      n4567 = Insert Into Array(array=w6615, index (row)=0 ("索引 (行)"), new element=w6639) -> (w6628:string[][])  [unwired: 1 in]
                    }
                    frame #1 {
                      n4568 = control-ref of="一级故障(从板)"() -> (w6655:refnum<vi>)
                      n4569 = property class="Clust (严格)"(reference=w6655) -> ("Value"=w6654:T15)  [unwired: 1 in, 2 out]
                      n4570 = Unbundle(w6654) -> ("电压过高"=w6653:dbl, "电压过低"=w6652:dbl, "温度过高"=w6651:dbl, "温度过低"=w6650:dbl, "电压不均衡(V)"=w6649:dbl, "温度不均衡"=w6648:dbl, "SOC过低"=w6647:dbl)
                      n4571 = Build Array(w6653, w6652, w6651, w6650, w6649, w6648, w6647) -> (w6646:dbl[])
                      n4572 = for {
                        tunnel: w6646 -> [w6657] mode=indexing
                        tunnel: [w6656] -> w6644 mode=indexing
                        n4573 = Format Into String(format string="%#f" ("格式字符串"), w6657) -> (resulting string=w6656:string)  [unwired: 2 in, 1 out]
                      }
                    }
                    frame #2 {
                      n4574 = control-ref of="二级故障(从板)"() -> (w6661:refnum<vi>)
                      n4575 = property class="Clust (严格)"(reference=w6661) -> ("Value"=w6670:T15)  [unwired: 1 in, 2 out]
                      n4576 = Unbundle(w6670) -> ("电压过高"=w6669:dbl, "电压过低"=w6668:dbl, "温度过高"=w6667:dbl, "温度过低"=w6666:dbl, "电压不均衡(V)"=w6665:dbl, "温度不均衡"=w6664:dbl, "SOC过低"=w6663:dbl)
                      n4577 = Build Array(w6669, w6668, w6667, w6666, w6665, w6664, w6663) -> (w6662:dbl[])
                      n4578 = for {
                        tunnel: w6662 -> [w6672] mode=indexing
                        tunnel: [w6671] -> w6659 mode=indexing
                        n4579 = Format Into String(format string="%#f" ("格式字符串"), w6672) -> (resulting string=w6671:string)  [unwired: 2 in, 1 out]
                      }
                    }
                    frame #3 {
                      n4580 = control-ref of="三级故障(从板)"() -> (w6685:refnum<vi>)
                      n4581 = property class="Clust (严格)"(reference=w6685) -> ("Value"=w6695:T15)  [unwired: 1 in, 2 out]
                      n4582 = Unbundle(w6695) -> ("电压过高"=w6694:dbl, "电压过低"=w6693:dbl, "温度过高"=w6692:dbl, "温度过低"=w6691:dbl, "电压不均衡(V)"=w6690:dbl, "温度不均衡"=w6689:dbl, "SOC过低"=w6688:dbl)
                      n4583 = Build Array(w6694, w6693, w6692, w6691, w6690, w6689, w6688) -> (w6687:dbl[])
                      n4584 = for {
                        tunnel: w6687 -> [w6697] mode=indexing
                        tunnel: [w6696] -> w6676 mode=indexing
                        n4585 = Format Into String(format string="%#f" ("格式字符串"), w6697) -> (resulting string=w6696:string)  [unwired: 2 in, 1 out]
                      }
                      n4586 = Insert Into Array(array=w6683, new element #1=w6682, new element #2=w6681, new element #3=string[] ["电压过高三级", "电压过低三级", "温度过高三级", "温度过低三级", "电压不均衡三级", "温度不均衡三级", "SOC过低三级"]) -> (w6674:string[])  [unwired: 1 in]
                      n4587 = Insert Into Array(array=w6679, new element #1=w6678, new element #2=w6677, new element #3=w6676) -> (w6675:string[])  [unwired: 1 in]
                      n4588 = Build Array(w6674, w6675) -> (w6686:string[][])
                      n4589 = Transpose 2D Array(2D array=w6686) -> (transposed array=w6684:string[][])
                    }
                    frame #4 {
                      n4590 = control-ref of="快换(从板)"() -> (w6721:refnum<vi>)
                      n4591 = property class="Clust (严格)"(reference=w6721) -> ("Value"=w6734:T16)  [unwired: 1 in, 2 out]
                      n4592 = Unbundle(w6734) -> ("串联数"=w6733:dbl, "并联数"=w6732:dbl, "电池厂家"=w6731:dbl, "电池类型"=w6730:dbl, "额定能量"=w6729:dbl, "额定容量"=w6728:dbl, "实际容量"=w6727:dbl, "额定总压"=w6720:dbl, "产权标识"=w6719:dbl, "应用车型"=w6718:dbl, "电池包组号"=w6717:dbl, "SOC"=w6715:dbl, "充电总安时"=w6714:dbl, "放电总安时"=w6713:dbl, "放空次数"=w6712:dbl, "充满次数"=w6711:dbl, "充电次数"=w6710:dbl, "车牌号"=w6700:string, "生产日期"=w6699:string, "最大允许单体电压"=w6709:dbl, "最大允许总电压"=w6708:dbl, "最大允许温度"=w6707:dbl, "最小允许温度"=w6706:dbl, "最大允许充电电流"=w6705:dbl, "最小允许充电电流"=w6704:dbl, "最小允许单体电压"=w6703:dbl, "电流步长"=w6702:dbl, "电池包序号"=w6701:dbl)
                      n4593 = Build Array(w6733, w6732, w6731, w6730, w6729, w6728, w6727, w6720, w6719, w6718, w6717, w6715, w6714, w6713, w6712, w6711, w6710, w6709, w6708, w6707, w6706, w6705, w6704, w6703, w6702, w6701) -> (w6726:dbl[])
                      n4594 = for {
                        tunnel: w6726 -> [w6736] mode=indexing
                        tunnel: [w6735] -> w6724 mode=indexing
                        n4595 = Format Into String(format string="%#f" ("格式字符串"), w6736) -> (resulting string=w6735:string)  [unwired: 2 in, 1 out]
                      }
                      n4596 = Insert Into Array(array=w6724, new element #1=w6700, new element #2=w6699) -> (w6716:string[])  [unwired: 1 in]
                      n4597 = call <vilib>:"Unset Busy.vi"() -> ()  [unwired: 2 in, 10 out]
                      n4598 = Build Array(string[] ["电池串联数", "电池并联数", "电池厂家", "额定能量", "额定容量", "实际容量", "额定总压", "产权标识", "应用车型", "电池包组号", "SOC", "充电总安时", "放电总安时", "放空次数", "充满次数", "充电次数", "最大允许单体电压", "最大允许总电压", "最大允许温度", "最小允许温度", "最大允许充电电流", "最小允许充电电流", "最小允许单体电压", "电流步长", "电池包序号"], w6716) -> (w6725:string[][])
                      n4599 = Transpose 2D Array(2D array=w6725) -> (transposed array=w6722:string[][])
                    }
                    frame #5 {
                      n4600 = local read "均衡参数"() -> (w6757:T17)
                      n4601 = Unbundle(w6757) -> ("充电结束电压(90%)"=w6749:sgl, "充电结束电压(91%)"=w6748:sgl, "充电结束电压(92%)"=w6747:sgl, "充电结束电压(93%)"=w6746:sgl, "充电结束电压(94%)"=w6745:sgl, "均衡计算-电压高阀值1级"=w6756:sgl, "均衡计算-电压高阀值2级"=w6755:sgl, "均衡计算-电压低阀值1级"=w6754:sgl, "均衡计算-电压低阀值2级"=w6753:sgl, "均衡计算-最低电压阀值"=w6752:sgl, "均衡停止-最低电压阀值"=w6751:sgl, "均衡计算-电压极差阀值"=w6750:sgl, "充电结束电压(95%)"=w6744:sgl, "充电结束电压(96%)"=w6743:sgl, "充电结束电压(97%)"=w6742:sgl, "充电结束电压(98%)"=w6741:sgl, "充电结束电压(99%)"=w6740:sgl, "充电结束电压(100%)"=w6739:sgl)
                      n4602 = Build Array(w6756, w6755, w6754, w6753, w6752, w6751, w6750, w6749, w6748, w6747, w6746, w6745, w6744, w6743, w6742, w6741, w6740, w6739) -> (w6761:sgl[])
                      n4603 = for {
                        tunnel: w6761 -> [w6763] mode=indexing
                        tunnel: [w6762] -> w6738 mode=indexing
                        n4604 = Format Into String(format string="%#f" ("格式字符串"), w6763) -> (resulting string=w6762:string)  [unwired: 2 in, 1 out]
                      }
                      n4605 = call <vilib>:"Unset Busy.vi"() -> ()  [unwired: 2 in, 10 out]
                      n4606 = Build Array(string[] ["均衡计算-电压高阀值1级", "均衡计算-电压高阀值2级", "均衡计算-电压低阀值1级", "均衡计算-电压低阀值2级", "均衡计算-最低电压阀值", "均衡停止-最低电压阀值", "均衡计算-电压极差阀值", "充电结束电压(90%)", "充电结束电压(91%)", "充电结束电压(92%)", "充电结束电压(93%)", "充电结束电压(94%)", "充电结束电压(95%)", "充电结束电压(96%)", "充电结束电压(97%)", "充电结束电压(98%)", "充电结束电压(99%)", "充电结束电压(100%)"], w6738) -> (w6760:string[][])
                      n4607 = Transpose 2D Array(2D array=w6760) -> (transposed array=w6758:string[][])
                    }
                  }
                  n4608 = Insert Into Array(array=w6607, index (col)=2 ("禁用的索引 (列)"), new element #1=w6605, new element #2=w6604) -> (w6606:string[][])  [unwired: 1 in]
                }
              }
              n4609 = call "当前时间解析-8.6.vi"() -> ("名称格式时间"=w6398:string)  [unwired: 1 in, 18 out]
              n4610 = Concatenate Strings(w6398, w6397) -> (w6395:string)
              n4611 = call <vilib>:"Application Directory.vi"() -> ("Application Directory"=w6392:path)
              n4612 = call "文件对话框2"("start path"=w6392, "prompt"="选择保存的路径", "default name"=w6395) -> ("selected path"=w6393:path, "cancelled"=w6391:bool, "error out"=w6390:errorcluster)  [unwired: 9 in, 1 out]
              n4613 = call <vilib>:"Clear Errors.vi"("error in (no error)"=w6390) -> ()  [unwired: 6 in, 1 out]
              n4614 = case shown="假" w6391 {
                tunnel: w6399 -> [w6404 _]
                tunnel: w6393 -> [w6400 _]
                frame False {
                  n4615 = call-poly <vilib>:"Write To Spreadsheet File.vi"("append to file? (new file:F)"=FALSE, "2D data"=w6404, "file path (dialog if empty)"=w6400) -> ("new file path (Not A Path if cancelled)"=w6402:path)  [unwired: 3 in, 2 out]
                  n4616 = Path To String(path=w6402) -> (string=w6401:string)
                  n4617 = stacked-sequence {
                    tunnel: w6401 -> [w6407]
                    frame #0 {
                      n4618 = Concatenate Strings("保存完成,路径为:" ("字符串"), w6407) -> (w6408:string)
                      n4619 = One Button Dialog(message=w6408, button name ("OK")="是" ("按钮名称（“确定”）")) -> ()  [unwired: 1 out]
                    }
                  }
                }
                frame True {
                }
              }
            }
            frame Disabled {
              n4620 = stacked-sequence {
                seq-local: [w6778] -> [_]
                frame #0 {
                  n4621 = local read "项目信息"() -> (w6780:string[][])
                  n4622 = local read "项目信息2"() -> (w6777:T9)
                  n4623 = Array Subset(array=w6780, index (row)=0 ("索引"), index (col)=0 ("索引"), length (col)=2 ("索引")) -> (w6783:string[][])  [unwired: 1 in]
                  n4624 = local read "一级故障"() -> ()  [unwired: 1 out]
                  n4625 = local read "从板个数"() -> (w6778:dbl)
                  n4626 = Unbundle(w6777) -> ("电池额定容量(A)"=w6776:dbl, "电池实际容量(A)"=w6775:dbl, "车架(牌)号"=w6769:string, "配置文件版本"=w6768:string, "SOH(%)"=w6773:dbl, "SOC(%)"=w6774:dbl, "产品编号"=w6770:string)  [unwired: 2 out]
                  n4627 = Index Array(array=w6783, index (col) #1=1 ("禁用的索引 (列)"), index (col) #2=0 ("索引 (列)")) -> (element #1=w6767:string[], element #2=w6766:string[])  [unwired: 2 in]
                  n4628 = Build Array(w6776, w6775, w6774, w6773) -> (w6772:dbl[])
                  n4629 = Number To Decimal String(number=w6778) -> ()  [unwired: 1 in, 1 out]
                  n4630 = for {
                    tunnel: w6772 -> [w6788] mode=indexing
                    tunnel: [w6787] -> w6771 mode=indexing
                    n4631 = Format Into String(format string="%#f" ("格式字符串"), w6788) -> (resulting string=w6787:string)  [unwired: 2 in, 1 out]
                  }
                  n4632 = Insert Into Array(array=w6771, new element #1=w6770, new element #2=w6769, new element #3=w6768, new element #4=w6767) -> ()  [unwired: 1 in, 1 out]
                  n4633 = Insert Into Array(array=string[] ["电池额定容量", "电池实际容量", "SOC", "SOH", "产品编号", "车架(牌)号", "配置文件版本"], new element=w6766) -> ()  [unwired: 1 in, 1 out]
                }
              }
            }
          }
        }
        frame "读配置文件" {
        }
      }
    }
    frame Error {
    }
  }
  n4634 = Release Queue(queue=w42, force destroy? (F)=TRUE ("强制销毁？(F)"), error in (no error)=w41) -> (error out=w44:errorcluster)  [unwired: 2 out]
  n4635 = call <vilib>:"Clear Errors.vi"("error in (no error)"=w44) -> ()  [unwired: 7 out]
  n4636 = local write "面板选择"(T7."读写参数" ("面板选择")) -> ()
  "失败?" <- FALSE
